vi "global_sub.vi"   [LabVIEW 2018]
uses:
  global.vi
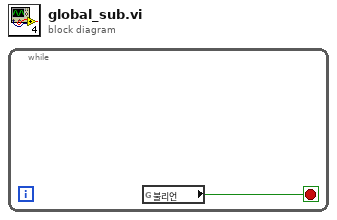
[diagram p0: block diagram]
diagram:
  n1 = while {
    stop <- w1 stop-if-true
    n2 = global read "global.vi" "불리언"() -> (w1:bool)
  }
